vi "YeeOffset.vi"(1 "file size (bytes)":i32, 2 "new file path":path) -> (0 "Numeric":i32)   [LabVIEW 2022 SP3]
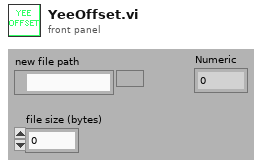
[diagram p1: front panel]
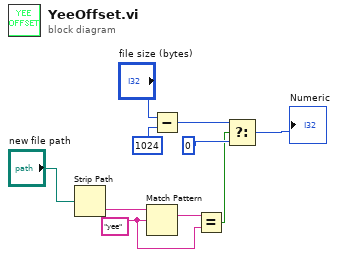
[diagram p0: block diagram]
diagram:
  w4 = "yee"
  n1 = Strip Path(path="new file path") -> (name=w2:string)  [unwired: 1 out]
  n2 = Match Pattern(string=w2, regular expression=w4) -> (match substring=w3:string)  [unwired: 4 out]
  n3 = Subtract(x="file size (bytes)", y=1024) -> (x-y=w9:i32)
  n4 = Equal?(x=w3, y=w4) -> (x = y?=w7:bool)
  n5 = Select(t=w9, s=w7, f=0) -> (s? t:f=→"Numeric":i32)
